vi "PID 1.vi"(8 "error in (no error)":errorcluster, 11 "State in":T1={"State"=enum."Idle", "Start Time"=timestamp(0 s since 1904-01-01), "Configuration"={"Cycle Period"=0.0, "Ismatech"={"VISA resource name"="", "Simulated?"=FALSE, "Pump Number"=1.0, "Reverse?"=FALSE}, "Masterflex"={"VISA resource name"="", "Simulated?"=FALSE, "Pump Number"=1.0, "Reverse?"=FALSE}, "Mettler"={"VISA resource name"="", "Simulated?"=FALSE}, "Bronkhorst M13 Flow Meter"={"VISA resource name"="", "Simulated?"=FALSE}, "PID 2 Parameters"={"Input Device"=enum."Bronkhorst M13", "Output Device"=enum."Ismatec ISM 831C", "Setpoint"=0.0, "PID gains"={"proportional gain (Kc)"=1.0, "integral time (Ti, min)"=0.01, "derivative time (Td, min)"=0.0}}, "Manual Entry"=0.0, "Auto?"=TRUE, "output range"={"output high"=100.0, "output low"=0.0}, "Bronkhorst M14"={"VISA resource name"="", "Simulated?"=FALSE}, "Tacmina Settings"={"Analog DAQ Task"="", "Digital DAQ Task"=""}, "KNF SIMDOS Settings"={"VISA resource name"="", "Simulated?"=TRUE}, "ASIA Pump C"={"ASIA Pump #"=0, "channel"=0, "Simulated"=FALSE}, "VICI Settings"={"VISA resource name"="", "Simulated?"=FALSE, "Pump Letter"="", "Reverse?"=FALSE}, "FLOM Settings"={"VISA resource name"="", "Simulated?"=TRUE, "Pump Number"=0.0}, "SSI PR Settings"={"VISA resource name"="", "Simulated?"=FALSE}}, "Current Time"=timestamp(0 s since 1904-01-01), "PID 1 Parameters"={"Setpoint"=0.0, "PID gains"={"proportional gain (Kc)"=1.0, "integral time (Ti, min)"=0.01, "derivative time (Td, min)"=0.0}}, "First Iteration"=FALSE, "Data"={"Flowmeter Output"=0.0, "Density"=0.0, "FL Temp"=0.0, "Scale Output (g)"=0.0, "Scale Rate of Change (g/min)"=0.0, "PID 1 Output"=0.0, "PID 2 Process Variable"=0.0, "PID 2 output"=0.0, "Pump Flow"=0.0, "Pump Pressure"=0.0}, "Process Name"="", "Pump On?"=enum."Off", "Input Error"=FALSE, "Output Error"=FALSE, "Log Started"=FALSE, "Current Setpoint"=0.0} {"PID 1 Parameters"."PID gains"."derivative time (Td, min)" format="%.3f"; "PID 1 Parameters"."PID gains"."integral time (Ti, min)" format="%.3f"; "PID 1 Parameters"."PID gains"."proportional gain (Kc)" format="%.3f"; "Configuration"."output range"."output low" min=0.0 max=100.0 format="%.2f"; "Configuration"."output range"."output high" format="%.2f"; "Configuration"."PID 2 Parameters"."PID gains"."derivative time (Td, min)" format="%.3f"; "Configuration"."PID 2 Parameters"."PID gains"."integral time (Ti, min)" format="%.3f"; "Configuration"."PID 2 Parameters"."PID gains"."proportional gain (Kc)" format="%.3f"; "Configuration"."ASIA Pump C"."channel" min=0 max=1 step=1; "Configuration"."Ismatech"."Pump Number" min=1.0 max=20.0 step=1.0; "Configuration"."Masterflex"."Pump Number" min=1.0 max=20.0 step=1.0}) -> (0 "error out":errorcluster, 3 "State out":T1={"State"=enum."Idle", "Start Time"=timestamp(0 s since 1904-01-01), "Configuration"={"Cycle Period"=0.0, "Ismatech"={"VISA resource name"="", "Simulated?"=FALSE, "Pump Number"=1.0, "Reverse?"=FALSE}, "Masterflex"={"VISA resource name"="", "Simulated?"=FALSE, "Pump Number"=1.0, "Reverse?"=FALSE}, "Mettler"={"VISA resource name"="", "Simulated?"=FALSE}, "Bronkhorst M13 Flow Meter"={"VISA resource name"="", "Simulated?"=FALSE}, "PID 2 Parameters"={"Input Device"=enum."Bronkhorst M13", "Output Device"=enum."Ismatec ISM 831C", "Setpoint"=0.0, "PID gains"={"proportional gain (Kc)"=1.0, "integral time (Ti, min)"=0.01, "derivative time (Td, min)"=0.0}}, "Manual Entry"=0.0, "Auto?"=TRUE, "output range"={"output high"=100.0, "output low"=0.0}, "Bronkhorst M14"={"VISA resource name"="", "Simulated?"=FALSE}, "Tacmina Settings"={"Analog DAQ Task"="", "Digital DAQ Task"=""}, "KNF SIMDOS Settings"={"VISA resource name"="", "Simulated?"=TRUE}, "ASIA Pump C"={"ASIA Pump #"=0, "channel"=0, "Simulated"=FALSE}, "VICI Settings"={"VISA resource name"="", "Simulated?"=FALSE, "Pump Letter"="", "Reverse?"=FALSE}, "FLOM Settings"={"VISA resource name"="", "Simulated?"=TRUE, "Pump Number"=0.0}, "SSI PR Settings"={"VISA resource name"="", "Simulated?"=FALSE}}, "Current Time"=timestamp(0 s since 1904-01-01), "PID 1 Parameters"={"Setpoint"=0.0, "PID gains"={"proportional gain (Kc)"=1.0, "integral time (Ti, min)"=0.01, "derivative time (Td, min)"=0.0}}, "First Iteration"=FALSE, "Data"={"Flowmeter Output"=0.0, "Density"=0.0, "FL Temp"=0.0, "Scale Output (g)"=0.0, "Scale Rate of Change (g/min)"=0.0, "PID 1 Output"=0.0, "PID 2 Process Variable"=0.0, "PID 2 output"=0.0, "Pump Flow"=0.0, "Pump Pressure"=0.0}, "Process Name"="", "Pump On?"=enum."Off", "Input Error"=FALSE, "Output Error"=FALSE, "Log Started"=FALSE, "Current Setpoint"=0.0} {"PID 1 Parameters"."PID gains"."derivative time (Td, min)" format="%.3f"; "PID 1 Parameters"."PID gains"."integral time (Ti, min)" format="%.3f"; "PID 1 Parameters"."PID gains"."proportional gain (Kc)" format="%.3f"; "Configuration"."output range"."output low" min=0.0 max=100.0 format="%.2f"; "Configuration"."output range"."output high" format="%.2f"; "Configuration"."PID 2 Parameters"."PID gains"."derivative time (Td, min)" format="%.3f"; "Configuration"."PID 2 Parameters"."PID gains"."integral time (Ti, min)" format="%.3f"; "Configuration"."PID 2 Parameters"."PID gains"."proportional gain (Kc)" format="%.3f"; "Configuration"."ASIA Pump C"."channel" min=0 max=1 step=1; "Configuration"."Ismatech"."Pump Number" min=1.0 max=20.0 step=1.0; "Configuration"."Masterflex"."Pump Number" min=1.0 max=20.0 step=1.0})   [LabVIEW 2018, in "Feed Module.lvlib" / "Feed Module Engine.lvlib"]
uses:
  Feed Module Engine.lvlib
  State Cluster.ctl
  State Enum.ctl
  Feed Module/Controls/Feed Module Settings Cluster.ctl
  Ismatec ISM 831C/Controls/Ismatech Settings Cluster.ctl
  Masterflex 7550-30/Controls/Settings Cluster.ctl
  Mettler Toledo/Controls/Settings Cluster.ctl
  Bronkhorst M13 Flow Meter/Settings Cluster.ctl
  PID 2 Parameters Cluster.ctl
  PID Input Enum.ctl
  PID 2 Output Enum.ctl
  Tacmina QI/Tacmina QI DAQ Setting.ctl
  KNF Pump/Settings Cluster plus SIMDOS.ctl
  ASIA Pump/Pump Settings.ctl
  VICI M50 Party Mode/Settings Cluster.ctl
  FLOM Pump/Settings Cluster.ctl
  SSI PR Class/SSI PR Settings Cluster.ctl
  PID 1 Parameters Cluster.ctl
  <vilib>/addons/control/pid/pid.llb/PID (DBL).vi
  <vilib>/addons/control/pid/NI_PID_pid.lvlib
  Feed Module/Feed Module.lvlib
  Ismatec ISM 831C/Ismatec ISM 831C.lvlib
  Masterflex 7550-30/Masterflex 7550-30.lvlib
  Mettler Toledo/Mettler Toledo.lvlib
  Bronkhorst M13 Flow Meter/Bronkhorst M13 Flow Meter.lvlib
  Tacmina QI/Tacmina QI.lvlib
  KNF Pump/KNF SIMDOS.lvlib
  ASIA Pump.lvlib
  VICI M50 Party Mode/VICI M6 M50 Party Mode.lvlib
  FLOM Pump/FLOM Pump.lvlib
  SSI PR Class/SSI PR Pump.lvlib
panel:
  # "Output Instruments"
  # "Input Instruments"
  # "Output Instruments"
  # "Input Instruments"
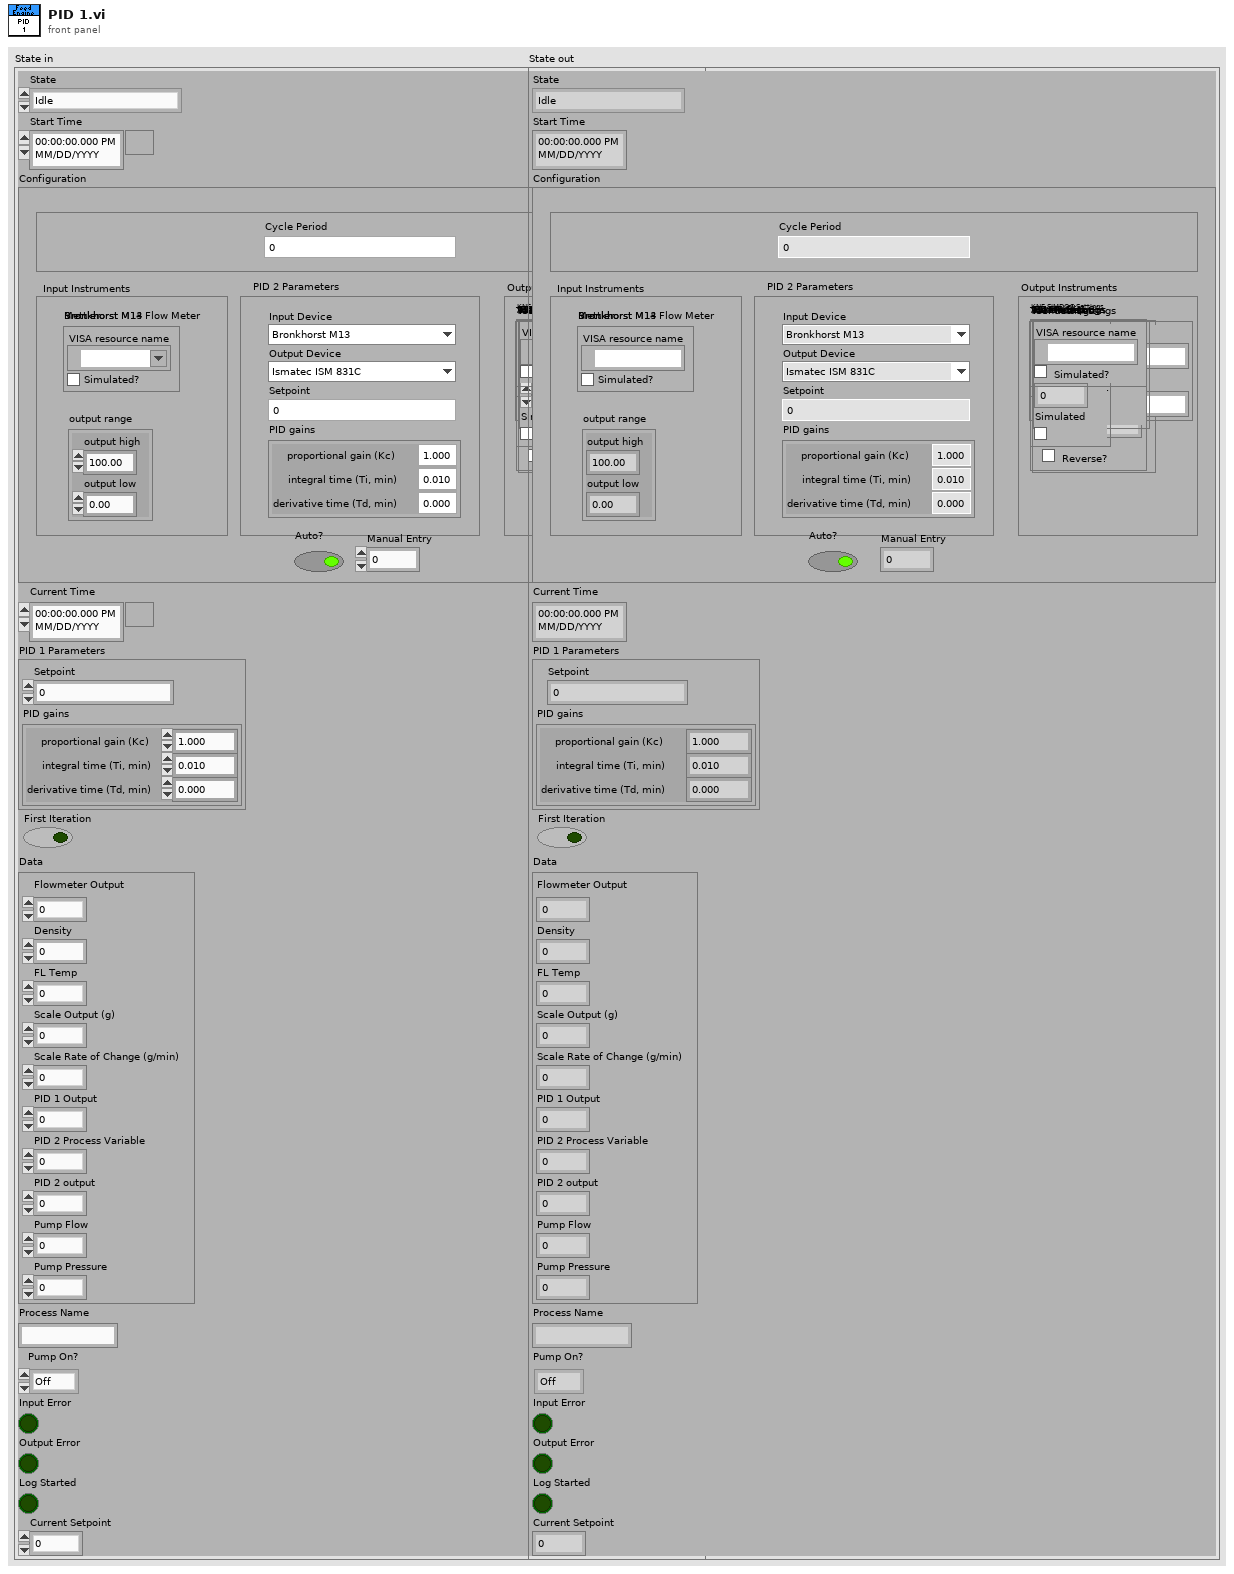
[diagram p1: front panel]
types:
  T1 = typedef "Feed Module.lvlib/Feed Module Engine.lvlib/State Cluster.ctl" = cluster{"State":T2, "Start Time":timestamp, "Configuration":T3, "Current Time":timestamp, "PID 1 Parameters":T17, "First Iteration":bool, "Data":cluster{"Flowmeter Output":dbl, "Density":dbl, "FL Temp":dbl, "Scale Output (g)":dbl, "Scale Rate of Change (g/min)":dbl, "PID 1 Output":dbl, "PID 2 Process Variable":dbl, "PID 2 output":dbl, "Pump Flow":dbl, "Pump Pressure":dbl}, "Process Name":string, "Pump On?":enum16{"Off", "On", "Not Initialized"}, "Input Error":bool, "Output Error":bool, "Log Started":bool, "Current Setpoint":dbl}
  T2 = typedef "Feed Module.lvlib/Feed Module Engine.lvlib/State Enum.ctl" = enum16{"Measuring", "Idle", "Paused"}
  T3 = typedef "Feed Module.lvlib/Feed Module Settings Cluster.ctl" = cluster{"Cycle Period":dbl, "Ismatech":T4, "Masterflex":T5, "Mettler":T6, "Bronkhorst M13 Flow Meter":T7, "PID 2 Parameters":T8, "Manual Entry":dbl, "Auto?":bool, "output range":cluster{"output high":dbl, "output low":dbl}, "Bronkhorst M14":T6, "Tacmina Settings":T11, "KNF SIMDOS Settings":T12, "ASIA Pump C":T13, "VICI Settings":T14, "FLOM Settings":T15, "SSI PR Settings":T16}
  T4 = typedef "Ismatec ISM 831C.lvlib/Ismatech Settings Cluster.ctl" = cluster{"VISA resource name":refnum<visa-resource-name>, "Simulated?":bool, "Pump Number":dbl, "Reverse?":bool}
  T5 = typedef "Masterflex 7550-30.lvlib/Settings Cluster.ctl" = cluster{"VISA resource name":refnum<visa-resource-name>, "Simulated?":bool, "Pump Number":dbl, "Reverse?":bool}
  T6 = typedef "Mettler Toledo.lvlib/Settings Cluster.ctl" = cluster{"VISA resource name":refnum<visa-resource-name>, "Simulated?":bool}
  T7 = typedef "Bronkhorst M13 Flow Meter.lvlib/Settings Cluster.ctl" = cluster{"VISA resource name":refnum<visa-resource-name>, "Simulated?":bool}
  T8 = typedef "PID 2 Parameters Cluster.ctl" = cluster{"Input Device":T9, "Output Device":T10, "Setpoint":dbl, "PID gains":cluster{"proportional gain (Kc)":dbl, "integral time (Ti, min)":dbl, "derivative time (Td, min)":dbl}}
  T9 = typedef "PID Input Enum.ctl" = enum16{"Default", "Bronkhorst M13", "Bronkhorst M14", "Scale Rate of Change"}
  T10 = typedef "PID 2 Output Enum.ctl" = enum16{"Default", "Ismatec ISM 831C", "Masterflex 7550-30", "VICI", "Tacmina QI", "KNF SIMDOS", "ASIA Type C", "FLOM UI-22-11", "SSI PR"}
  T11 = typedef "Tacmina QI.lvlib/Tacmina QI DAQ Setting.ctl" = cluster{"Analog DAQ Task":refnum<k21>, "Digital DAQ Task":refnum<k21>}
  T12 = typedef "KNF SIMDOS.lvlib/Settings Cluster plus SIMDOS.ctl" = cluster{"VISA resource name":refnum<visa-resource-name>, "Simulated?":bool}
  T13 = typedef "ASIA Pump.lvlib/Pump Settings.ctl" = cluster{"ASIA Pump #":i32, "channel":i32, "Simulated":bool}
  T14 = typedef "VICI M6 M50 Party Mode.lvlib/Settings Cluster.ctl" = cluster{"VISA resource name":refnum<visa-resource-name>, "Simulated?":bool, "Pump Letter":string, "Reverse?":bool}
  T15 = typedef "FLOM Pump.lvlib/Settings Cluster.ctl" = cluster{"VISA resource name":refnum<visa-resource-name>, "Simulated?":bool, "Pump Number":dbl}
  T16 = typedef "SSI PR Pump.lvlib/SSI PR Settings Cluster.ctl" = cluster{"VISA resource name":refnum<visa-resource-name>, "Simulated?":bool}
  T17 = typedef "PID 1 Parameters Cluster.ctl" = cluster{"Setpoint":dbl, "PID gains":cluster{"proportional gain (Kc)":dbl, "integral time (Ti, min)":dbl, "derivative time (Td, min)":dbl}}
  T18 = cluster{"proportional gain (Kc)":dbl, "integral time (Ti, min)":dbl, "derivative time (Td, min)":dbl}
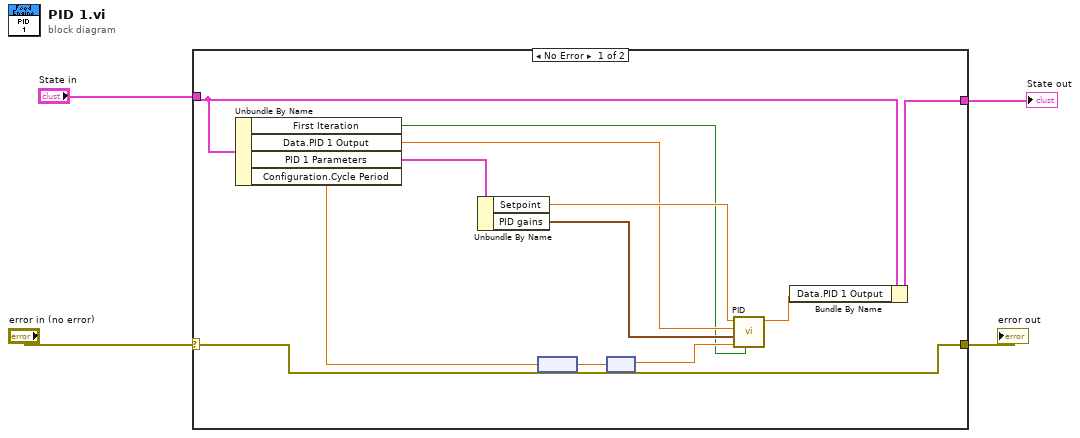
[diagram p0: block diagram]
diagram:
  n1 = case shown="No Error" "error in (no error)" {
    selector: "error in (no error)" -> [w12 w18]
    tunnel: [w12 w18] -> w3
    tunnel: "State in" -> [w9 w17]
    tunnel: [w10 w17] -> w1
    frame No Error {
      n2 = Unbundle By Name(w9) -> ("First Iteration"=w5:bool, "Data.PID 1 Output"=w7:dbl, "PID 1 Parameters"=w8:T17, "Configuration.Cycle Period"=w6:dbl)
      n3 = Unbundle By Name(w8) -> ("Setpoint"=w16:dbl, "PID gains"=w15:T18)
      n4 = node(w6) -> (w14:dbl[unit])
      n5 = node(w14) -> (w13:dbl)
      n6 = call-poly <vilib>:"PID.vi"("reinitialize? (F)"=w5, "dt (s)"=w13, "PID gains"=w15, "process variable"=w7, "setpoint"=w16) -> ("output"=w11:dbl)  [unwired: 5 in, 1 out]
      n7 = Bundle By Name(cluster=w9, "Data.PID 1 Output"=w11) -> (w10:T1)
    }
    frame Error {
    }
  }
  "error out" <- w3
  "State out" <- w1
